vi "linkdin doc.vi"() -> ()   [LabVIEW 2020]
panel:
  in  "stop":bool
  in  "i/p":bool
  out "o/p":i32
  in  "B":i32
  in  "A":i32
  in  "stop":bool
  out "LED":bool
  in  "Press":bool
  out "Deg F":dbl
  in  "Deg C":dbl
  in  "stop":bool
  in  "OK Button":bool
  out "o/p":dbl
  in  "i/p":dbl
  out "o/p":dbl
  in  "X1":dbl
  in  "X2":dbl
  in  "Y1":dbl
  in  "Y2":dbl
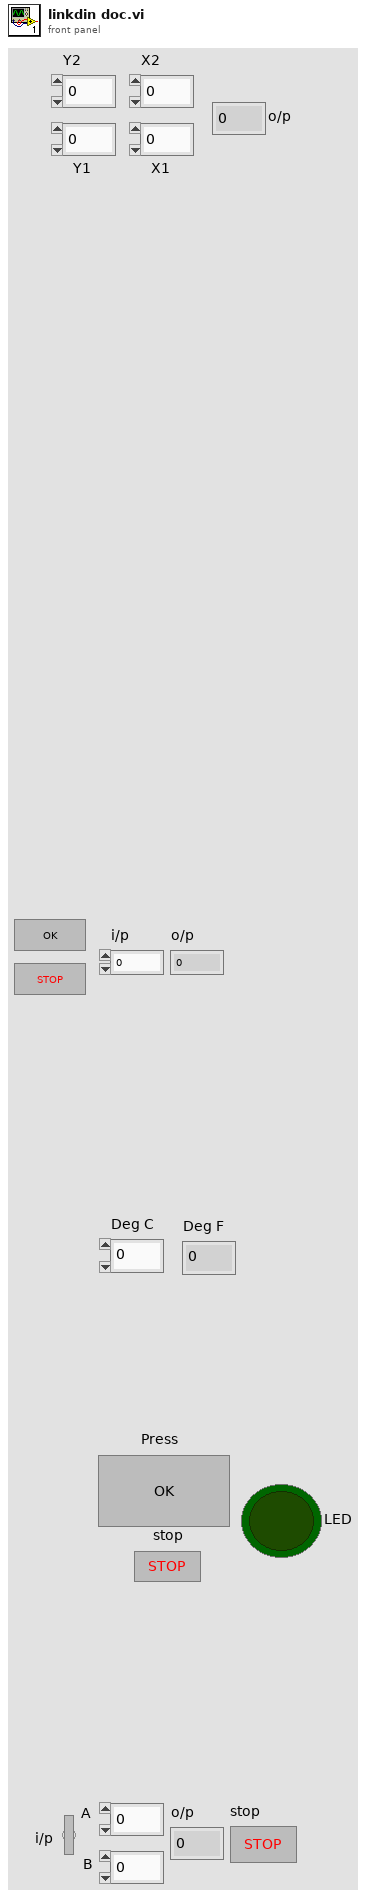
[diagram p1: front panel]
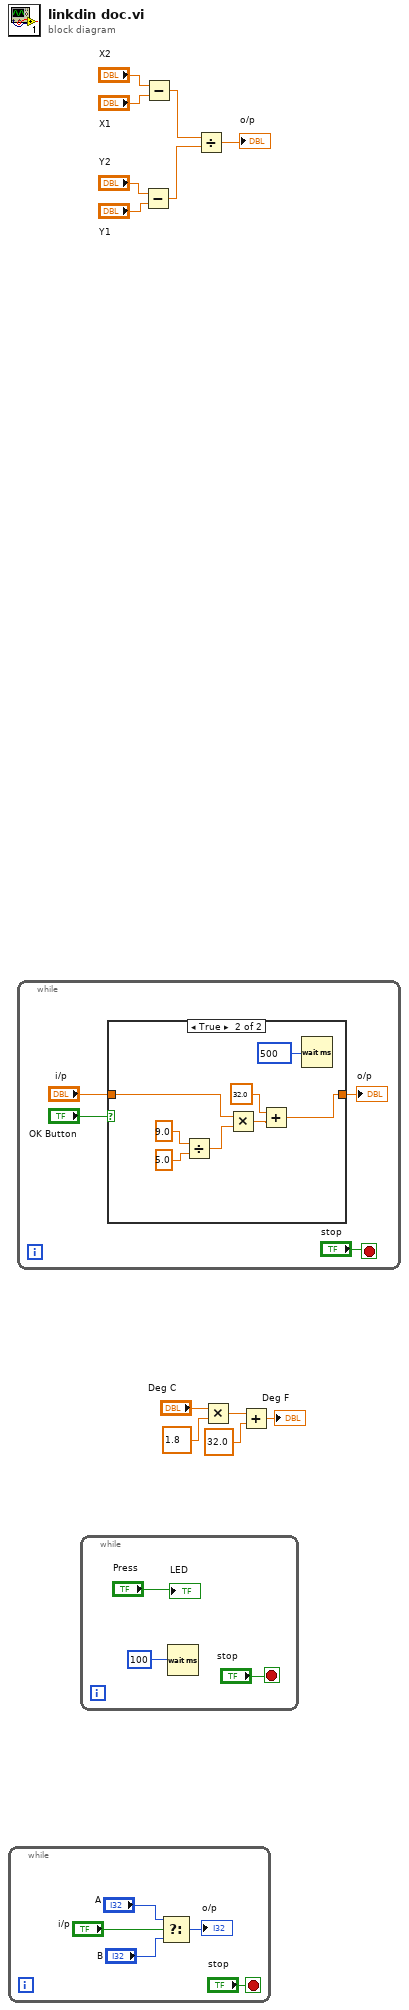
[diagram p0: block diagram]
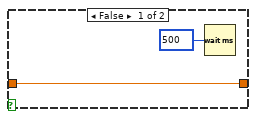
[diagram p2: hidden frame]
diagram:
  n1 = while {
    stop <- "stop" stop-if-true
    n2 = Select(t="A", s="i/p", f="B") -> (s? t:f=→"o/p":i32)
  }
  n3 = while {
    stop <- "stop" stop-if-true
    n4 = case shown="True" "OK Button" {
      tunnel: "i/p" -> [w23 w26]
      tunnel: [w23 w25] -> w19
      frame False {
        n5 = Wait (ms)(milliseconds to wait=u32 500 ("millisecond timer value")) -> ()  [unwired: 1 out]
      }
      frame True {
        n6 = Divide(x=9.0, y=5.0) -> (x/y=w29:dbl)
        n7 = Multiply(x=w26, y=w29) -> (x*y=w28:dbl)
        n8 = Add(x=32.0, y=w28) -> (x+y=w25:dbl)
        n9 = Wait (ms)(milliseconds to wait=u32 500 ("millisecond timer value")) -> ()  [unwired: 1 out]
      }
    }
    "o/p" <- w19
  }
  n10 = while {
    stop <- "stop" stop-if-true
    n11 = Wait (ms)(milliseconds to wait=u32 100 ("millisecond timer value")) -> ()  [unwired: 1 out]
    "LED" <- "Press"
  }
  n12 = Subtract(x="Y2", y="Y1") -> (x-y=w8:dbl)
  n13 = Subtract(x="X2", y="X1") -> (x-y=w7:dbl)
  n14 = Divide(x=w7, y=w8) -> (x/y=→"o/p":dbl)
  n15 = Multiply(x="Deg C", y=1.8) -> (x*y=w1:dbl)
  n16 = Add(x=w1, y=32.0) -> (x+y=→"Deg F":dbl)
